vi "_MDPtr DecrementCount.vi"(9 "error in (no error)":errorcluster, 10 "HexStrPtr":T1) -> (1 "String Attribute":string, 2 "error out":errorcluster, 3 "HexStrPtr (dup)":T1)   [LabVIEW 2017, in "MDPtr.lvlib"]
uses:
  MDPtr.lvlib
  MDPtr TypeDef/MDPtr.ctl
  MDPtr TypeDef/MDPtr DataFrame-Memory.ctl
  MDPtr TypeDef/MDPtr DataFrame-Common.ctl
  <vilib>/Utility/Data Type/Type Definitions/Data Type.ctl
  _MDPtr Build Error Cluster.vi
  <vilib>/Utility/Data Type/NI_Data Type.lvlib
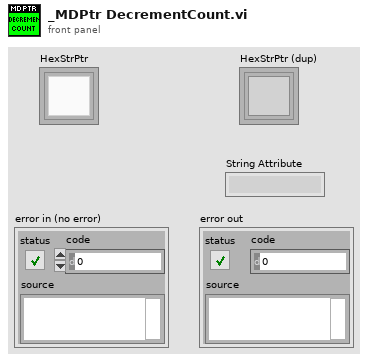
[diagram p1: front panel]
types:
  T1 = typedef "MDPtr.lvlib/MDPtr.ctl" = refnum<k1>
  T2 = typedef "MDPtr.lvlib/MDPtr DataFrame-Memory.ctl" = cluster{"Common":T3, "DVR":refnum<data-value>}
  T3 = typedef "MDPtr.lvlib/MDPtr DataFrame-Common.ctl" = cluster{"Data Type":T4, "Copy Count":i32, "String Attribute":string, "Cache Length":i32, "Data Length":i32}
  T4 = typedef "NI_Data Type.lvlib/Data Type.ctl" = enum8{"Invalid Type", "Void", "I8", "I16", "I32", "I64", "U8", "U16", "U32", "U64", "Single Float", "Double Float", "Extended Float", "Single Complex", "Double Complex", "Extended Complex", "Enum U8", "Enum U16", "Enum U32", "Enum U64", "Single Float With Unit", "Double Float With Unit", "Extended Float With Unit", "Single Complex with Unit", "Double Complex with Unit", "Extended Complex with Unit", "Boolean", "String", "Path", "Picture", "Tag", "Array", "Cluster", "Variant", "LV Variant", "Waveform", "Timestamp", "Digital Waveform", "Digital Data", "ExpressData", "Refnum", "External Data", "VI", "Poly VI", "LabVIEW Class Instance", "Fixed Point"}
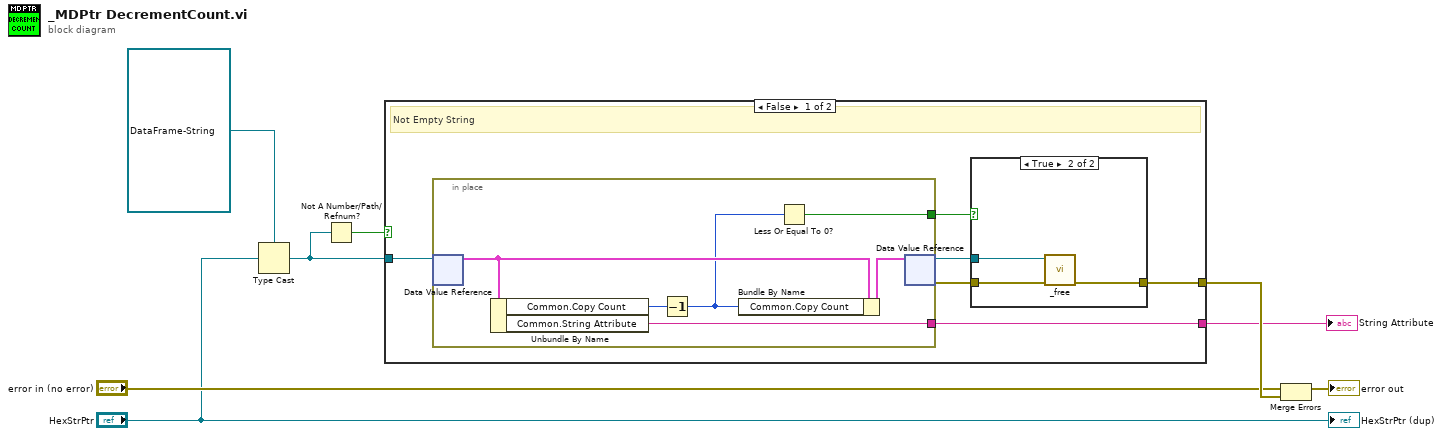
[diagram p0: block diagram]
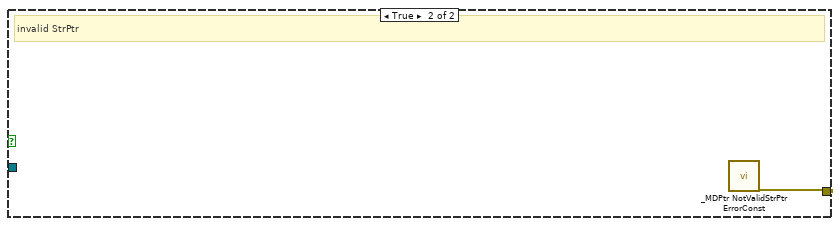
[diagram p3: hidden frame]
diagram:
  n1 = Type Cast(type=refnum<data-value> refnum ("data value reference"), x="HexStrPtr") -> (*(type *) &x=w2:refnum<data-value>)
  n2 = Not A Number/Path/Refnum?(number/path/refnum=w2) -> (NaN/Path/Refnum?=w3:bool)
  n3 = case shown="False" w3 {
    tunnel: [w12 w25] -> w8
    tunnel: w2 -> [w13 _]
    tunnel: [w9 _] -> w1
    frame False {
      # "Not Empty String"
      n4 = in-place {
        in-place-border: [w20] -> w10
        in-place-border: [w19] -> w9
        n5 = in-place-dvr #1(w13) -> (w23:T2)  [unwired: 1 out]
        n6 = Unbundle By Name(w23) -> ("Common.Copy Count"=w22:i32, "Common.String Attribute"=w19:string)
        n7 = Decrement(x=w22) -> (x-1=w21:i32)
        n8 = Bundle By Name(cluster=w23, "Common.Copy Count"=w21) -> (w24:T2)
        n9 = Less Or Equal To 0?(x=w21) -> (x <= 0?=w20:bool)
        n10 = in-place-dvr #1(w24) -> (w11:refnum<data-value>, w14:errorcluster)
      }
      n11 = case shown="True" w10 {
        tunnel: w14 -> [w15 w18]
        tunnel: [w15 w17] -> w12
        tunnel: w11 -> [_ w16]
        frame False {
        }
        frame True {
          n12 = call "_free.vi"("error in (no error)"=w18, "MDPtr DVR"=w16) -> ("error out"=w17:errorcluster)  [unwired: 8 in]
        }
      }
    }
    frame True {
      # "invalid StrPtr"
      n13 = call "_MDPtr NotValidStrPtr ErrorConst.vi"() -> ("error out"=w25:errorcluster)  [unwired: 19 in]
    }
  }
  "String Attribute" <- w1
  n14 = Merge Errors("error in (no error)", w8) -> (→"error out":errorcluster)
  "HexStrPtr (dup)" <- "HexStrPtr"
